vi "KGN Get Pump Concentrations.vi"(7 "scaling":dbl=1000000.0, 8 "Fehler (Eingang, kein Fehler)":errorcluster, 9 "Info Cluster":T2, 10 "VISA-Ressourcenname":refnum<visa-resource-name>, 11 "device (Eingang)":u32) -> (0 "Fehler (Ausgang)":errorcluster, 1 "Info Cluster out":T2, 2 "VISA-Ressourcenname out":refnum<visa-resource-name>, 3 "dup device (Ausgang)":u32, 4 "Pump Concentrations-Cluster":T1(array[cluster]), 6 "Kommandos gesendet":string)   [LabVIEW 2020, in "Linearisierung v2.lvlib" / "Gasteiler.lvlib" / "HovaCAL_Interface.lvlib" / "KGN.lvlib" / "KGN GUI Get.lvlib"]
uses:
  KGN GUI Get.lvlib
  Controls/Info Cluster.ctl
  get/get.lvlib
  Controls/Controls.lvlib
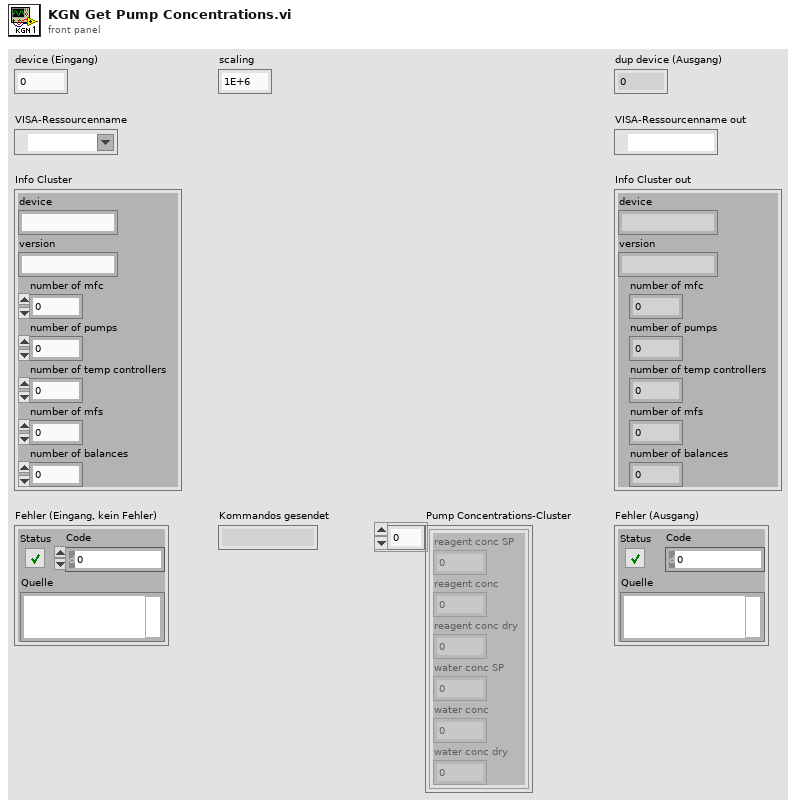
[diagram p1: front panel]
types:
  T1 = cluster{"reagent conc SP":dbl, "reagent conc":dbl, "reagent conc dry":dbl, "water conc SP":dbl, "water conc":dbl, "water conc dry":dbl}[]
  T2 = typedef "Linearisierung v2.lvlib/Gasteiler.lvlib/HovaCAL_Interface.lvlib/Controls.lvlib/Info Cluster.ctl" = cluster{"device":string, "version":string, "number of mfc":i32, "number of pumps":i32, "number of temp controllers":i32, "number of mfs":i32, "number of balances":i32}
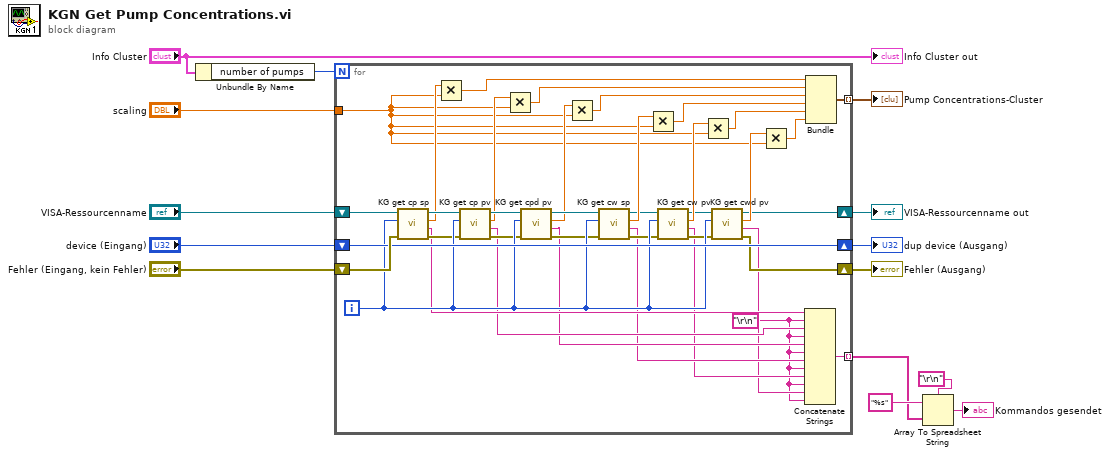
[diagram p0: block diagram]
diagram:
  n1 = Unbundle By Name("Info Cluster") -> ("number of pumps"=w8:i32)
  n2 = for {
    N: w8 -> [_]
    tunnel: [w51] -> w10 mode=indexing
    shift-right: [w50] -> w12
    shift-left: "device (Eingang)" -> [w50]
    shift-right: [w49] -> w11
    shift-left: "Fehler (Eingang, kein Fehler)" -> [w52]
    tunnel: "scaling" -> [w23]
    shift-right: [w40] -> w5
    shift-left: "VISA-Ressourcenname" -> [w41]
    tunnel: [w15] -> w2 mode=indexing
    i -> [w48]
    w16 = "\r\n"
    n3 = call "KG get cp sp.vi"("Fehler (Eingang, kein Fehler)"=w52, "pump"=w48, "VISA-Ressourcenname"=w41) -> ("Fehler (Ausgang)"=w39:errorcluster, "Kommando gesendet"=w22:string, "Concentration"=w24:dbl, "VISA-Ressourcenname (Ausgang)"=w34:refnum<visa-resource-name>)  [unwired: 5 in]
    n4 = Multiply(x=w24, y=w23) -> (x*y=w25:dbl)
    n5 = call "KG get cp pv.vi"("Fehler (Eingang, kein Fehler)"=w39, "pump"=w48, "VISA-Ressourcenname"=w34) -> ("Fehler (Ausgang)"=w38:errorcluster, "Kommando gesendet"=w21:string, "Concentration"=w26:dbl, "VISA-Ressourcenname (Ausgang)"=w33:refnum<visa-resource-name>)  [unwired: 5 in]
    n6 = Multiply(x=w26, y=w23) -> (x*y=w27:dbl)
    n7 = call "KG get cpd pv.vi"("Fehler (Eingang, kein Fehler)"=w38, "pump"=w48, "VISA-Ressourcenname"=w33) -> ("Fehler (Ausgang)"=w37:errorcluster, "Kommando gesendet"=w20:string, "Concentration"=w28:dbl, "VISA-Ressourcenname (Ausgang)"=w32:refnum<visa-resource-name>)  [unwired: 5 in]
    n8 = Multiply(x=w28, y=w23) -> (x*y=w29:dbl)
    n9 = call "KG get cw sp.vi"("Fehler (Eingang, kein Fehler)"=w37, "pump"=w48, "VISA-Ressourcenname"=w32) -> ("Fehler (Ausgang)"=w36:errorcluster, "Kommando gesendet"=w19:string, "Concentration"=w47:dbl, "VISA-Ressourcenname (Ausgang)"=w31:refnum<visa-resource-name>)  [unwired: 5 in]
    n10 = Multiply(x=w47, y=w23) -> (x*y=w46:dbl)
    n11 = call "KG get cw pv.vi"("Fehler (Eingang, kein Fehler)"=w36, "pump"=w48, "VISA-Ressourcenname"=w31) -> ("Fehler (Ausgang)"=w35:errorcluster, "Kommando gesendet"=w18:string, "Concentration"=w45:dbl, "VISA-Ressourcenname (Ausgang)"=w30:refnum<visa-resource-name>)  [unwired: 5 in]
    n12 = Multiply(x=w45, y=w23) -> (x*y=w44:dbl)
    n13 = call "KG get cwd pv.vi"("Fehler (Eingang, kein Fehler)"=w35, "pump"=w48, "VISA-Ressourcenname"=w30) -> ("Fehler (Ausgang)"=w49:errorcluster, "Kommando gesendet"=w17:string, "Concentration"=w43:dbl, "VISA-Ressourcenname (Ausgang)"=w40:refnum<visa-resource-name>)  [unwired: 5 in]
    n14 = Multiply(x=w43, y=w23) -> (x*y=w42:dbl)
    n15 = Concatenate Strings(w22, w16, w21, w16, w20, w16, w19, w16, w18, w16, w17, w16) -> (w15:string)
    n16 = Bundle(w25, w27, w29, w46, w44, w42) -> (w51:cluster{dbl, dbl, dbl, dbl, dbl, dbl})  [unwired: 1 in]
  }
  "dup device (Ausgang)" <- w12
  "Fehler (Ausgang)" <- w11
  "Pump Concentrations-Cluster" <- w10
  "VISA-Ressourcenname out" <- w5
  n17 = Array To Spreadsheet String(delimiter (Tab)="\r\n", array=w2, 3:"%s" ("Format-String")) -> (spreadsheet string=→"Kommandos gesendet":string)
  "Info Cluster out" <- "Info Cluster"
